vi "Create Ellipse Mask.vi"() -> ()   [LabVIEW 2012, in "Picture Box Tools.lvlib"]
uses:
  Picture Box Tools.lvlib
  <vilib>/picture/picture.llb/imagedata.ctl
  Rectangle Tools/Rect/Rect Tools.lvlib
panel:
  out "Mask Picture":picture
  out "picture":picture caption="Picture"
  out "Masked picture":picture caption="Masked Picture"
  in  "color(black)":u32(colorbox) caption="颜色（黑色）"
  in  "image data":T1={"image type"=0, "image depth"=24, "image"=array[49050 elements], "mask"=[], "colors"=[], "Rectangle"={"left"=0, "top"=0, "right"=109, "bottom"=150}} caption="图像数据"
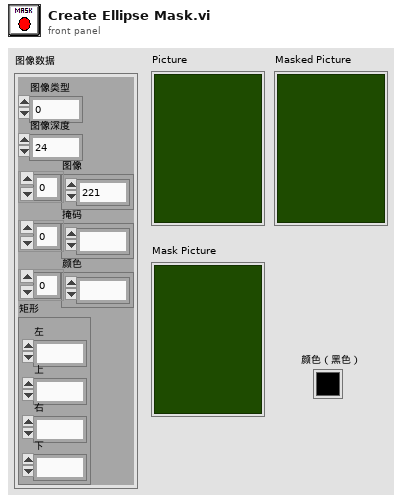
[diagram p1: front panel]
types:
  T1 = typedef "imagedata.ctl" = cluster{"image type":i32, "image depth":i32, "image":u8[], "mask":u8[], "colors":u32[], "Rectangle":cluster{"left":i16, "top":i16, "right":i16, "bottom":i16}}
  T2 = cluster{"left":i16, "top":i16, "right":i16, "bottom":i16}
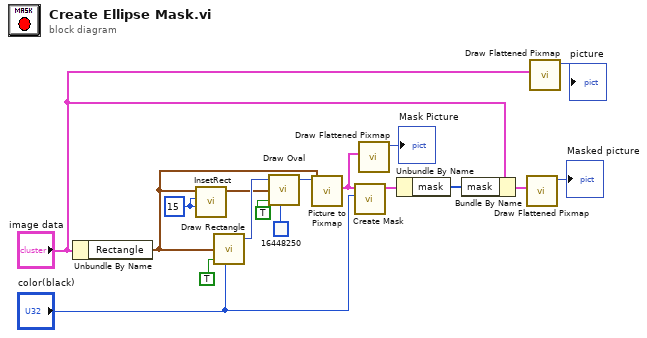
[diagram p0: block diagram]
diagram:
  w8 = i16 15 ("dh")
  n1 = Unbundle By Name("image data") -> ("Rectangle"=w12:T2)
  n2 = call "InsetRect.vi"("dv"=w8, "dh"=w8, "rect"=w12) -> ("inset rect"=w7:T2)  [unwired: 7 in, 1 out]
  n3 = call <vilib>:"Draw Rectangle.vi"("rect"=w12, "fill?(F)"=TRUE, "color(black)"="color(black)") -> ("new picture"=w16:picture)  [unwired: 6 in]
  n4 = call <vilib>:"Draw Oval.vi"("picture"=w16, "rect"=w7, "fill?(F)"=TRUE, "color(black)"=u32 16448250) -> ("new picture"=w13:picture)  [unwired: 5 in]
  n5 = call <vilib>:"Picture to Pixmap.vi"("rect"=w12, "picture"=w13) -> ("image data"=w3:T1)  [unwired: 8 in, 1 out]
  n6 = call <vilib>:"Create Mask.vi"("Mask Color (Black)"="color(black)", "image data"=w3) -> ("image data"=w11:T1)  [unwired: 9 in]
  n7 = call <vilib>:"Draw Flattened Pixmap.vi"("image data"=w3) -> ("new picture"=→"Mask Picture":picture)  [unwired: 8 in]
  n8 = Unbundle By Name(w11) -> ("mask"=w10:u8[])
  n9 = Bundle By Name(cluster="image data", "mask"=w10) -> (w9:T1)
  n10 = call <vilib>:"Draw Flattened Pixmap.vi"("image data"=w9) -> ("new picture"=→"Masked picture":picture)  [unwired: 8 in]
  n11 = call <vilib>:"Draw Flattened Pixmap.vi"("image data"="image data") -> ("new picture"=→"picture":picture)  [unwired: 8 in]
